vi "String to Multiline Attribute.vi"(8 "error in (no error)":errorcluster, 11 "Multiline String":string) -> (0 "error out":errorcluster, 3 "Multiline Attribute":string)   [LabVIEW 2019, in "NIPKG Packager.lvclass"]
doc: "Reformat a multiline string to be used as a multiline attribute for the NI Package Manager."
uses:
  NIPKG Packager.lvclass
  <vilib>/Utility/error.llb/whitespace.ctl
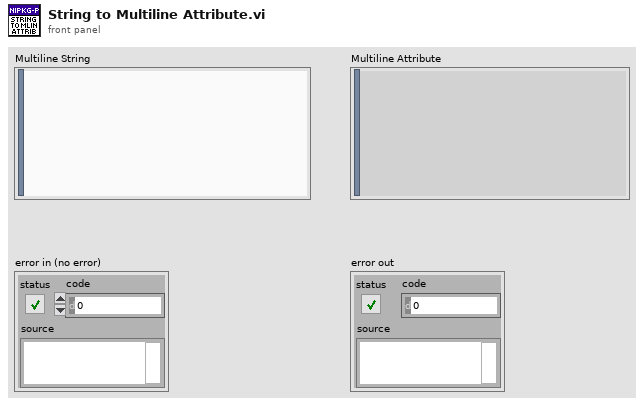
[diagram p1: front panel]
types:
  T1 = typedef "whitespace.ctl" = u16
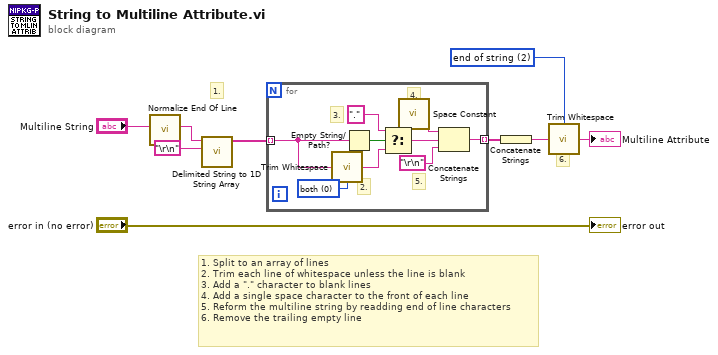
[diagram p0: block diagram]
diagram:
  w1 = T1 2 items=["both", "start of string", "end of string"] ("location (both)")
  # "6."
  # "1."
  # "1. Split to an array of lines\n2. Trim each line of whitespace unless the line is blank\n3. Add a \".\" character to blank lines\n4. Add a single space character to the front of each line\n5. Reform the multiline string by readding end of line characters\n6. Remove the trailing empty line"
  n1 = call <vilib>:"Normalize End Of Line.vi"("string in"="Multiline String") -> ("string out"=w7:string)  [unwired: 7 in]
  n2 = call <vilib>:"Delimited String to 1D String Array.vi"("delimiter"="\r\n", "delimited string"=w7) -> ("string array"=w5:string[])  [unwired: 9 in]
  n3 = for {
    tunnel: w5 -> [w17] mode=indexing
    tunnel: [w11] -> w4 mode=indexing
    w14 = T1 0 items=["both", "start of string", "end of string"] ("location (both)")
    # "5."
    # "4."
    # "2."
    # "3."
    n4 = call <vilib>:"Trim Whitespace.vi"("string"=w17, "location (both)"=w14) -> ("trimmed string"=w16:string)
    n5 = Empty String/Path?(string/path=w17) -> (empty?=w18:bool)
    n6 = Select(t=".", s=w18, f=w16) -> (s? t:f=w13:string)
    n7 = call <vilib>:"Space Constant.vi"() -> ("String"=w12:string)
    n8 = Concatenate Strings(w12, w13, "\r\n") -> (w11:string)
  }
  n9 = Concatenate Strings(w4) -> (w3:string)
  n10 = call <vilib>:"Trim Whitespace.vi"("string"=w3, "location (both)"=w1) -> ("trimmed string"=→"Multiline Attribute":string)
  "error out" <- "error in (no error)"
